vi "timetest4.vi"() -> ()   [LabVIEW 2015]
uses:
  BERTTA.dll
panel:
  out "element 6":i32
  out "return type":dbl
  in  "direction":i32
  in  "Tcurrent":dbl=20.0
  in  "Tset":dbl=100.0
  in  "rt":i32=600
  out "element 5":i32
  out "element 4":i32
  out "element 3":i32
  out "element 2":i32
  out "element":i32
  in  "pause":i32
  in  "start":i32
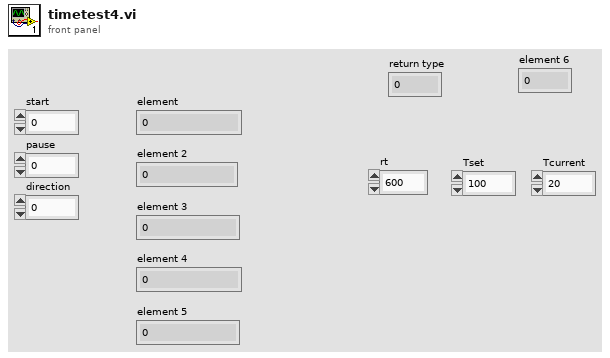
[diagram p1: front panel]
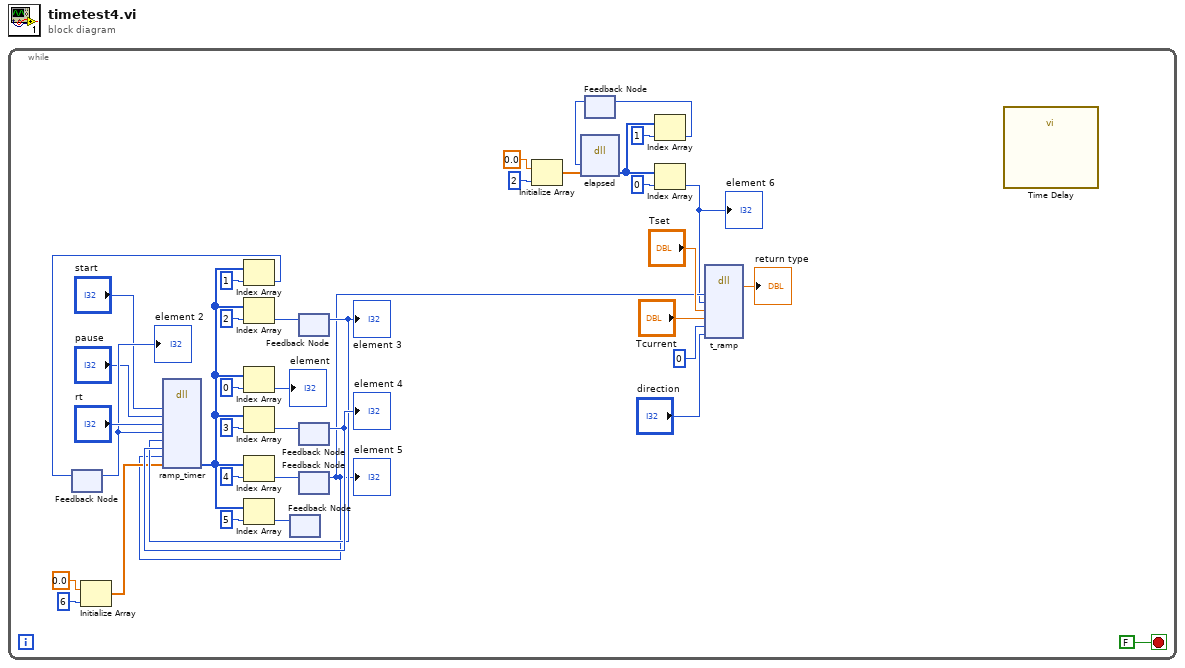
[diagram p0: block diagram]
diagram:
  n1 = while {
    stop <- FALSE stop-if-true
    n2 = feedback #1() -> (w22:i32)  [unwired: 1 in]
    "element 2" <- w22
    n3 = Initialize Array(0.0 ("element"), 6 ("dimension size")) -> (w14:dbl[])
    n4 = feedback #2() -> ()  [unwired: 2 in]
    n5 = feedback #3() -> (w24:i32)  [unwired: 1 in]
    "element 3" <- w24
    n6 = feedback #4() -> (w27:i32)  [unwired: 1 in]
    "element 4" <- w27
    n7 = feedback #5() -> (w11:i32)  [unwired: 1 in]
    "element 5" <- w11
    n8 = dll-call lib="C:/Users/xlaraser/Documents/Visual Studio 2017/Projects/Bertta/BERTTA/Debug/BERTTA.dll" fn="ramp_timer"("enable"="start", "pause"="pause", "rt"="rt", "start_time"=w22, "pause_time"=w24, "paused"=w27, "paused_old"=w11, "params"=w14) -> ("params"=w33:i32[])  [unwired: 11 in, 2 out]
    n9 = Index Array(array=w33, index=1) -> (element=w21:i32)
    n10 = feedback-in #1(w21) -> ()
    n11 = Index Array(array=w33, index=2) -> (element=w23:i32)
    n12 = Index Array(array=w33, index=0) -> (element=→"element":i32)
    n13 = Index Array(array=w33, index=3) -> (element=w26:i32)
    n14 = Index Array(array=w33, index=4) -> (element=w29:i32)
    n15 = Index Array(array=w33, index=5) -> (element=w32:i32)
    n16 = feedback-in #2(w32) -> ()
    n17 = feedback-in #3(w23) -> ()
    n18 = feedback-in #4(w26) -> ()
    n19 = feedback-in #5(w29) -> ()
    n20 = Initialize Array(0.0 ("element"), 2 ("dimension size")) -> (w10:dbl[])
    n21 = feedback #6() -> (w3:i32)  [unwired: 1 in]
    n22 = dll-call lib="C:/Users/xlaraser/Documents/Visual Studio 2017/Projects/Bertta/BERTTA/Debug/BERTTA.dll" fn="elapsed"("last_time"=w3, "params"=w10) -> ("params"=w6:i32[])  [unwired: 5 in, 2 out]
    n23 = Index Array(array=w6, index=1) -> (element=w4:i32)
    n24 = feedback-in #6(w4) -> ()
    n25 = Index Array(array=w6, index=0) -> (element=w2:i32)
    "element 6" <- w2
    n26 = dll-call lib="C:/Users/xlaraser/Documents/Visual Studio 2017/Projects/Bertta/BERTTA/Debug/BERTTA.dll" fn="t_ramp"("ramp_time"=w11, "elapsed"=w2, "Tset"="Tset", "Tcurrent"="Tcurrent", "rt"=0, "direction"="direction") -> ("return type"=→"return type":dbl)  [unwired: 9 in, 2 out]
    n27 = call "Time Delay"() -> ()  [unwired: 11 in, 1 out]
  }
